vi "findfirst0.vi"(11 "Array":i32[][](array[numeric])) -> (2 "index of element":i32)   [LabVIEW 2013]
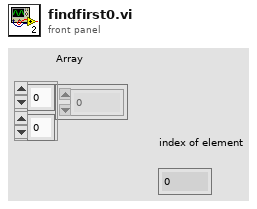
[diagram p1: front panel]
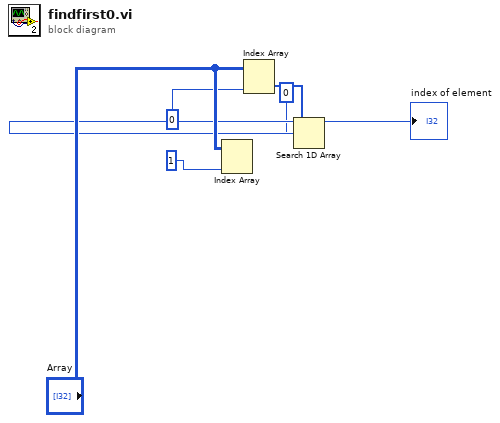
[diagram p0: block diagram]
diagram:
  n1 = Index Array(array="Array", index (col)=1) -> ()  [unwired: 1 in, 1 out]
  n2 = Index Array(array="Array", index (col)=0) -> (element=w3:i32[])  [unwired: 1 in]
  n3 = Search 1D Array(1D array=w3, element=0) -> (index of element=→"index of element":i32)  [unwired: 1 in]
